vi "UI_ShowIn_Subpanel.vi"(8 "error in (no error)":errorcluster, 10 "Sub Panel":refnum<vi>, 11 "D&C_SchemaBase in":refnum<class "D&C_SchemaBase.lvclass">) -> (0 "error out":errorcluster, 3 "D&C_SchemaBase out":refnum<class "D&C_SchemaBase.lvclass">)   [LabVIEW 2020, in "D&C_SchemaBase.lvlib" / "D&C_SchemaBase.lvclass"]
uses:
  D&C_SchemaBase.lvclass
  support/UI_Actor.lvlibp/UI_Actor/UI_Actor.lvclass
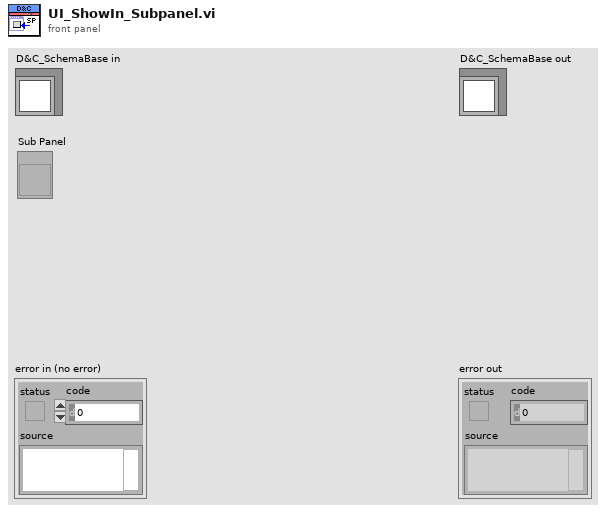
[diagram p1: front panel]
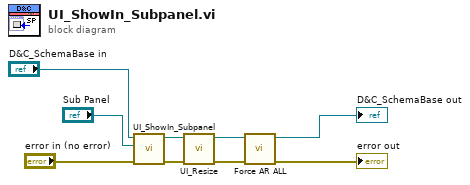
[diagram p0: block diagram]
diagram:
  n1 = call-parent "UI_ShowIn_Subpanel.vi"("error in (no error)"="error in (no error)", "Sub Panel"="Sub Panel", "UI_Actor in"="D&C_SchemaBase in") -> ("error out"=w6:errorcluster, "UI_Actor out"=w5:refnum<class "D&C_SchemaBase.lvclass">)  [unwired: 7 in]
  n2 = call-dynamic "UI_Resize.vi"("error in (no error)"=w6, "D&C_SchemaBase in"=w5) -> ("error out"=w3:errorcluster, "D&C_SchemaBase out"=w4:refnum<class "D&C_SchemaBase.lvclass">)  [unwired: 8 in]
  n3 = call "Force AR ALL.vi"("error in (no error)"=w3, "D&C_SchemaBase in"=w4) -> ("error out"=→"error out":errorcluster, "D&C_SchemaBase out"=→"D&C_SchemaBase out":refnum<class "D&C_SchemaBase.lvclass">)  [unwired: 8 in]
